vi "Grab.vi"(8 "error in (no error)":errorcluster, 11 "reference in":refnum<class "Camera_Sim.lvclass">) -> (0 "error out":errorcluster, 1 "Frame Number":u32, 2 "Image Out":T1, 3 "reference out":refnum<class "Camera_Sim.lvclass">)   [LabVIEW 2017, in "Camera_Sim.lvclass"]
doc: "Grabs the latest image in the image buffer for an acquisition that has been started. Must be used with Start and StopAcquisition."
uses:
  Camera_Sim.lvclass
  <vilib>/vision/Image Controls.llb/IMAQ Image.ctl
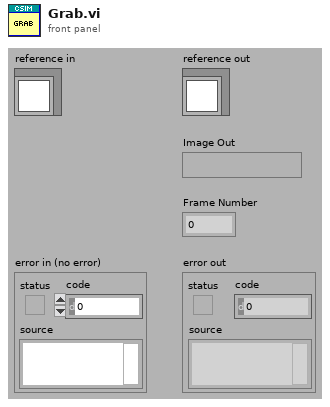
[diagram p1: front panel]
types:
  T1 = typedef "IMAQ Image.ctl" = refnum<image>
  T2 = typedef "Camera_Sim.lvclass/ObjectAttributes.ctl" = cluster{"Connected":bool, "Image Out":T1, "Frame Number":u32, "Image Directory":path, "Images in Directory":path[]}
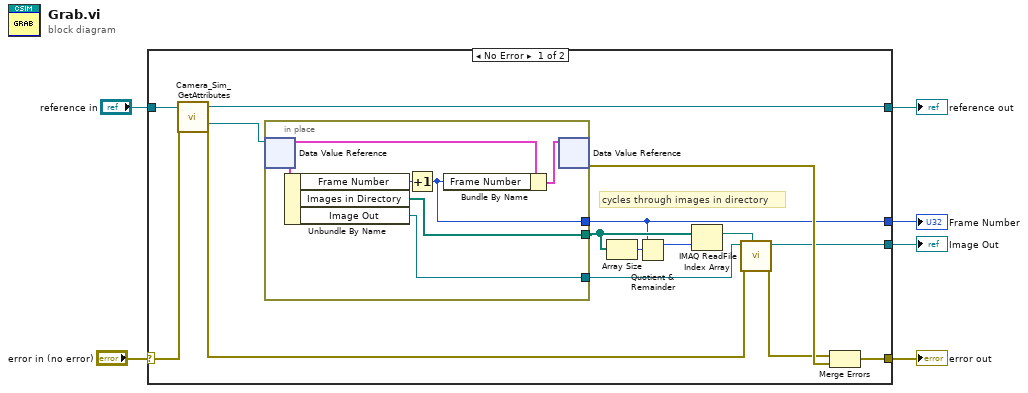
[diagram p0: block diagram]
diagram:
  n1 = case shown="No Error" "error in (no error)" {
    selector: "error in (no error)" -> [w19 w29]
    tunnel: [w16 w29] -> w5
    tunnel: [w20 w28] -> w3
    tunnel: "reference in" -> [w21 w28]
    tunnel: [w7 _] -> w2
    tunnel: [w13 _] -> w1
    frame No Error {
      # "cycles through images in directory"
      n2 = call "Camera_Sim_GetAttributes.vi"("reference in"=w21, "error in (no error)"=w19) -> ("reference out"=w20:refnum<class "Camera_Sim.lvclass">, "DataRef"=w17:refnum<data-value>, "error out"=w15:errorcluster)  [unwired: 10 in, 1 out]
      n3 = in-place {
        in-place-border: [w24] -> w7
        in-place-border: [w23] -> w12
        in-place-border: [w22] -> w11
        n4 = in-place-dvr #1(w17) -> (w27:T2)  [unwired: 1 out]
        n5 = Unbundle By Name(w27) -> ("Frame Number"=w25:u32, "Images in Directory"=w23:path[], "Image Out"=w22:T1)
        n6 = Increment(x=w25) -> (x+1=w24:u32)
        n7 = Bundle By Name(cluster=w27, "Frame Number"=w24) -> (w26:T2)
        n8 = in-place-dvr #1(w26) -> (w18:errorcluster)  [unwired: 1 out]
      }
      n9 = Array Size(array=w12) -> (size(s)=w8:i32)
      n10 = Quotient & Remainder(x=w7, y=w8) -> (x-y*floor(x/y)=w9:u32)  [unwired: 1 out]
      n11 = Index Array(array=w12, index=w9) -> (element=w10:path)
      n12 = call "IMAQ ReadFile"("File Path"=w10, "error in (no error)"=w15, "Image"=w11) -> ("error out"=w14:errorcluster, "Image Out"=w13:T1)  [unwired: 2 in, 5 out]
      n13 = Merge Errors(w14, w18) -> (w16:errorcluster)
    }
    frame Error {
    }
  }
  "error out" <- w5
  "reference out" <- w3
  "Frame Number" <- w2
  "Image Out" <- w1
